vi "encoderCalculations.vi"(10 "Right Distance In":dbl, 11 "Left Distance In":dbl) -> (2 "Right Ticks":dbl, 3 "Left Ticks":dbl)   [LabVIEW 2015]
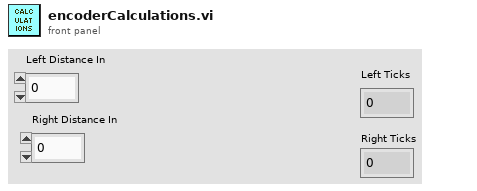
[diagram p1: front panel]
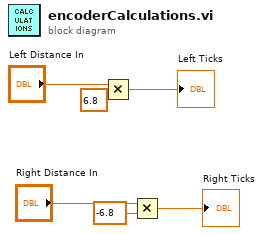
[diagram p0: block diagram]
diagram:
  n1 = Multiply(x="Left Distance In", y=6.8) -> (x*y=→"Left Ticks":dbl)
  n2 = Multiply(x="Right Distance In", y=-6.8) -> (x*y=→"Right Ticks":dbl)
